vi "Get Python Session.vi"(11 "Python Session in":refnum<k35>) -> (3 "Python Session out":refnum<k35>)   [LabVIEW 2023, in "LabVIEW AI Base.lvlib"]
uses:
  LabVIEW AI Base.lvlib
  AI Base Globals.vi
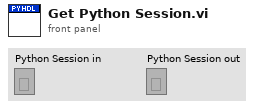
[diagram p1: front panel]
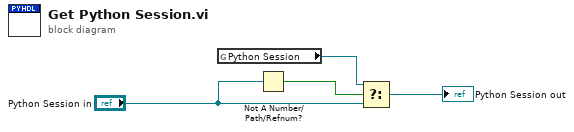
[diagram p0: block diagram]
diagram:
  n1 = global read "AI Base Globals.vi" "Python Session"() -> (w4:refnum<k35>)
  n2 = Not A Number/Path/Refnum?(number/path/refnum="Python Session in") -> (NaN/Path/Refnum?=w3:bool)
  n3 = Select(t=w4, s=w3, f="Python Session in") -> (s? t:f=→"Python Session out":refnum<k35>)
